vi "Write Scalings.vi"(8 "error in (no error)":errorcluster, 10 "Scalings":T1[](array[typedef]), 11 "Scaling in":refnum<class "Scaling.lvclass">) -> (0 "error out":errorcluster, 3 "Scaling out":refnum<class "Scaling.lvclass">)   [LabVIEW 2024, in "Scaling.lvclass"]
doc: "Scaling.lvclass:Write Scalings.vi\n\nThis VI overwrites the Scalings defined in the current configuration file's class data. The configuration must silll be written to disk for the Scalings to be saved.\n\nInstrument Communication Module Version 1.0\nNovember, 2017 Original Code Consulting David Thomson\n www.originalcode.com"
uses:
  Scaling.lvclass
  Scaling Def.ctl
  Scaling.lvclass/Scaling.ctl
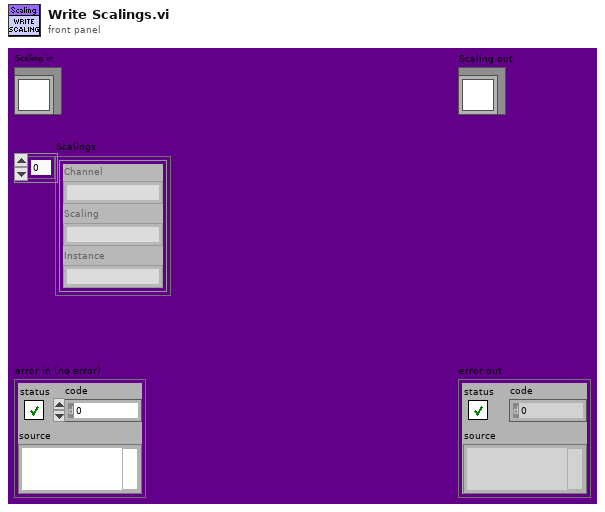
[diagram p1: front panel]
types:
  T1 = typedef "Scaling Def.ctl" = cluster{"Channel":string, "Scaling":string, "Instance":string}
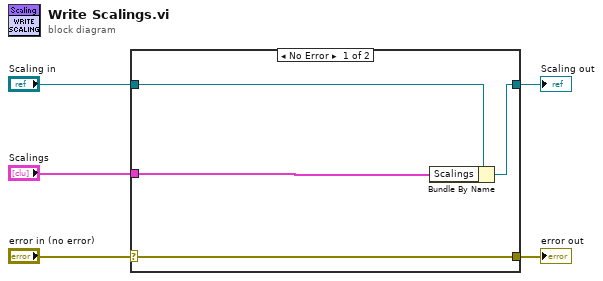
[diagram p0: block diagram]
diagram:
  n1 = case shown="No Error" "error in (no error)" {
    selector: "error in (no error)" -> [w9 w10]
    tunnel: [w9 w10] -> w4
    tunnel: [w7 w11] -> w2
    tunnel: "Scaling in" -> [w8 w11]
    tunnel: "Scalings" -> [w6 _]
    frame No Error {
      n2 = Bundle By Name(cluster=w8, "Scalings"=w6) -> (w7:refnum<class "Scaling.lvclass">)
    }
    frame Error {
    }
  }
  "error out" <- w4
  "Scaling out" <- w2
